vi "StartandConnectCore.vi"(8 "error in (no error)":errorcluster, 10 "Service Details":T1, 11 "MicronClient in":refnum<class "MicronClient.lvclass">) -> (0 "error out":errorcluster, 3 "MicronClient out":refnum<class "MicronClient.lvclass">)   [LabVIEW 2019, in "MicronClient.lvclass"]
uses:
  MicronClient.lvclass
  Typedefs/ServiceDetails.ctl
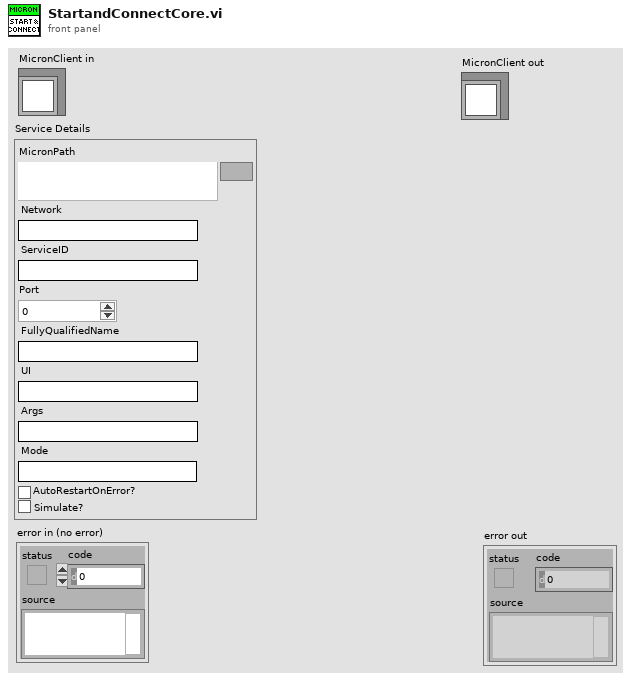
[diagram p1: front panel]
types:
  T1 = typedef "MicronClient.lvclass/ServiceDetails.ctl" = cluster{"MicronPath":path, "Network":string, "ServiceID":string, "Port":i32, "FullyQualifiedName":string, "UI":string, "Args":string, "Mode":string, "AutoRestartOnError?":bool, "Simulate?":bool}
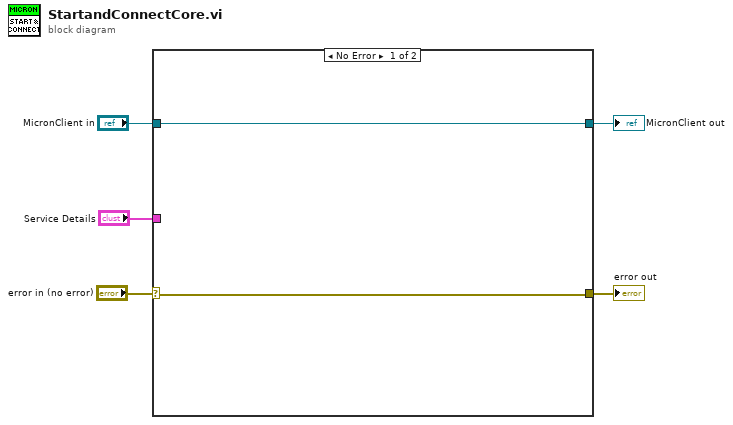
[diagram p0: block diagram]
diagram:
  n1 = case shown="No Error" "error in (no error)" {
    selector: "error in (no error)" -> [w6 w9]
    tunnel: [w6 w9] -> w4
    tunnel: [w7 w8] -> w2
    tunnel: "MicronClient in" -> [w7 w8]
    tunnel: "Service Details" -> [_ _]
    frame No Error {
    }
    frame Error {
    }
  }
  "error out" <- w4
  "MicronClient out" <- w2
